vi "Plugin Configuration.Initialize.vi"(8 "error in (no error)":errorcluster, 10 "Plugin Configuration cluster":T1={"name"="", "class"="", "cycle timing"={"priority"=0, "decimation"=1, "offset"=0}, "Transfer Groups"=[], "settings"=[]}, 11 "Plugin Configuration in":refnum<class "Plugin Configuration.lvclass">) -> (0 "error out":errorcluster, 3 "Plugin Configuration":refnum<class "Plugin Configuration.lvclass">)   [LabVIEW 2017, in "DSF Core.lvlib" / "Plugin Configuration.lvclass"]
uses:
  Plugin Configuration.lvclass
  C:/Git/DSF/Data Sharing Framework/Source/Core/Shared/Classes/Configuration/Configuration.lvclass
  DSF Configuration API/Public/Controls/DSF Engine Plugin Configuration.ctl
  DSF Configuration API/Public/Controls/DSF Timing Info.ctl
  DSF Configuration API/Public/Controls/DSF Engine Transfer Group Configuration.ctl
  DSF Configuration API/Public/Controls/DSF Direction.ctl
  DSF Configuration API/Public/Controls/DSF Engine Transfer Configuration.ctl
  DSF Configuration API/Public/Controls/DSF Byte Order.ctl
  DSF Configuration API/Public/Controls/DSF Engine Channel Configuration.ctl
  DSF Configuration API/Public/Controls/DSF Data Type.ctl
  DSF Configuration API/Public/Controls/DSF Settings Info.ctl
  Configuration/Configuration.lvclass/Configuration.ctl
  Plugin Configuration.lvclass/Plugin Configuration.ctl
  Transfer Group/Transfer Group Configuration.lvclass
  Configuration/Configuration.lvclass
  DSF Configuration.lvlib
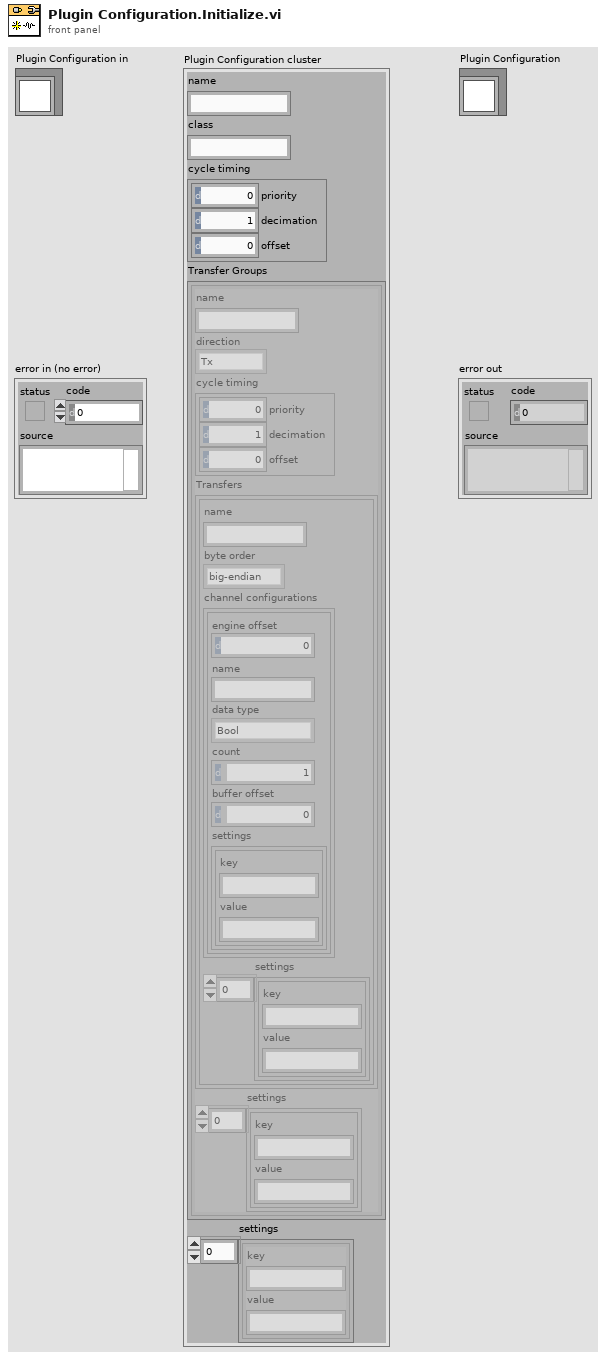
[diagram p1: front panel]
types:
  T1 = typedef "DSF Configuration.lvlib/DSF Engine Plugin Configuration.ctl" = cluster{"name":string, "class":string, "cycle timing":T2, "Transfer Groups":T3[], "settings":T9}
  T2 = typedef "DSF Configuration.lvlib/DSF Timing Info.ctl" = cluster{"priority":u64, "decimation":u64, "offset":u64}
  T3 = typedef "DSF Configuration.lvlib/DSF Engine Transfer Group Configuration.ctl" = cluster{"name":string, "direction":T4, "cycle timing":T2, "Transfers":T5[], "settings":T9}
  T4 = typedef "DSF Configuration.lvlib/DSF Direction.ctl" = enum8{"Tx", "Rx"}
  T5 = typedef "DSF Configuration.lvlib/DSF Engine Transfer Configuration.ctl" = cluster{"name":string, "byte order":T6, "channel configurations":T7[], "settings":T9}
  T6 = typedef "DSF Configuration.lvlib/DSF Byte Order.ctl" = enum8{"big-endian", "little-endian"}
  T7 = typedef "DSF Configuration.lvlib/DSF Engine Channel Configuration.ctl" = cluster{"engine offset":u64, "name":string, "data type":T8, "count":u64, "buffer offset":u64, "settings":T9}
  T8 = typedef "DSF Configuration.lvlib/DSF Data Type.ctl" = enum8{"Bool", "SGL", "DBL", "I8", "I16", "I32", "I64", "U8", "U16", "U32", "U64"}
  T9 = typedef "DSF Configuration.lvlib/DSF Settings Info.ctl" = cluster{"key":string, "value":string}[]
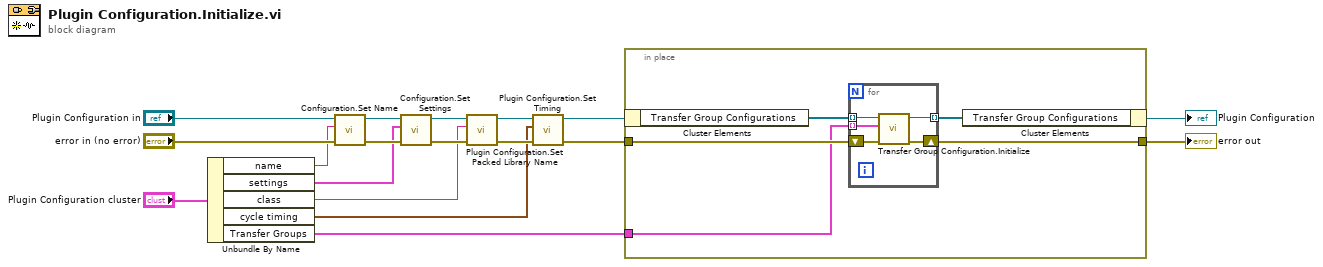
[diagram p0: block diagram]
diagram:
  n1 = Unbundle By Name("Plugin Configuration cluster") -> ("name"=w2:string, "settings"=w1:T9, "class"=w8:string, "cycle timing"=w7:T2, "Transfer Groups"=w6:T3[])
  n2 = call "Configuration.Set Name.vi"("name"=w2, "Configuration in"="Plugin Configuration in") -> ("Configuration out"=w4:refnum<class "Plugin Configuration.lvclass">)  [unwired: 9 in]
  n3 = call "Configuration.Set Settings.vi"("settings"=w1, "Configuration in"=w4) -> ("Configuration out"=w5:refnum<class "Plugin Configuration.lvclass">)  [unwired: 9 in]
  n4 = call "Plugin Configuration.Set Packed Library Name.vi"("packed library name"=w8, "Plugin Configuration in"=w5) -> ("Plugin Configuration out"=w13:refnum<class "Plugin Configuration.lvclass">)  [unwired: 9 in]
  n5 = call "Plugin Configuration.Set Timing.vi"("cycle timing"=w7, "Plugin Configuration in"=w13) -> ("Plugin Configuration out"=w12:refnum<class "Plugin Configuration.lvclass">)  [unwired: 9 in]
  n6 = in-place {
    in-place-border: "error in (no error)" -> [w17]
    in-place-border: [w16] -> w10
    in-place-border: w6 -> [w15]
    n7 = in-place-cluster #1(w12) -> ("Transfer Group Configurations"=w19:refnum<class "Transfer Group Configuration.lvclass">[])
    n8 = for {
      tunnel: w19 -> [w24] mode=indexing
      tunnel: [w23] -> w18 mode=indexing
      shift-right: [w22] -> w16
      shift-left: w17 -> [w21]
      tunnel: w15 -> [w20] mode=indexing
      n9 = call-dynamic "Transfer Group Configuration.Initialize.vi"("error in (no error)"=w21, "Transfer Group Configuration cluster"=w20, "Transfer Group Configuration in"=w24) -> ("error out"=w22:errorcluster, "Transfer Group Configuration"=w23:refnum<class "Transfer Group Configuration.lvclass">)  [unwired: 7 in]
    }
    n10 = in-place-cluster #1("Transfer Group Configurations"=w18) -> (→"Plugin Configuration":refnum<class "Plugin Configuration.lvclass">)
  }
  "error out" <- w10
